vi "Insert SubPanl.vi"(8 "error in (no error)":errorcluster, 10 "VI Ref":refnum<vi>, 11 "Subpanel Ref":refnum<vi>) -> (0 "error out":errorcluster)   [LabVIEW 2021, in "Model.lvlib"]
doc: "<b>Note:</b> This VI was modified by the <b>Validate DQMH Module</b> tool to turn off automatic error handling."
uses:
  Model/Model.lvlib
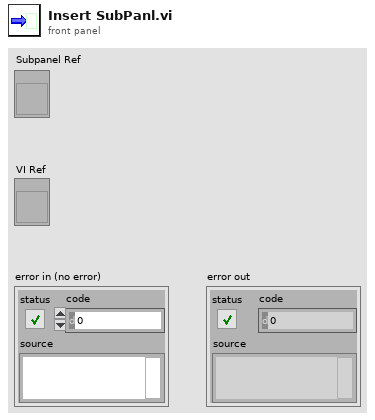
[diagram p1: front panel]
types:
  T1 = enum32{"Invalid", "Standard", "Closed", "Hidden", "Minimized", "Maximized"}
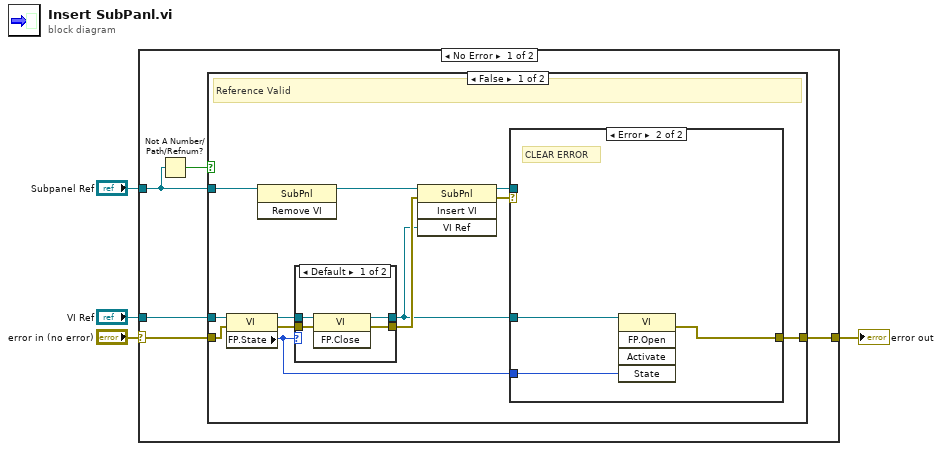
[diagram p0: block diagram]
diagram:
  n1 = case shown="No Error" "error in (no error)" {
    selector: "error in (no error)" -> [w8 w33]
    tunnel: "VI Ref" -> [w9 _]
    tunnel: "Subpanel Ref" -> [w5 _]
    tunnel: [w7 w33] -> w1
    frame No Error {
      n2 = Not A Number/Path/Refnum?(number/path/refnum=w5) -> (NaN/Path/Refnum?=w6:bool)
      n3 = case shown="False" w6 {
        tunnel: w9 -> [w21 _]
        tunnel: w8 -> [w13 w32]
        tunnel: [w12 w32] -> w7
        tunnel: w5 -> [w11 _]
        frame False {
          # "Reference Valid"
          n4 = property class="VI"(reference=w21, error in=w13) -> (reference out=w20:refnum<vi>, error out=w19:errorcluster, "FP.State"=w14:T1)
          n5 = invoke class="SubPnl" method="Remove VI"(reference=w11) -> (reference out=w10:refnum<vi>)  [unwired: 2 in, 2 out]
          n6 = case shown="Default" w14 {
            tunnel: w20 -> [w25 w27]
            tunnel: w19 -> [w24 w26]
            tunnel: [w23 w27] -> w15
            tunnel: [w22 w26] -> w18
            frame Default {
              n7 = invoke class="VI" method="FP.Close"(reference=w25, error in=w24) -> (reference out=w23:refnum<vi>, error out=w22:errorcluster)  [unwired: 1 in, 1 out]
            }
            frame "Closed" {
            }
          }
          n8 = invoke class="SubPnl" method="Insert VI"(reference=w10, error in=w18, "VI Ref"=w15) -> (reference out=w16:refnum<vi>, error out=w17:errorcluster)  [unwired: 1 in, 2 out]
          n9 = case shown="Error" w17 {
            selector: w17 -> [w28 _]
            tunnel: w16 -> [_ _]
            tunnel: w15 -> [_ w31]
            tunnel: w14 -> [_ w30]
            tunnel: [w28 w29] -> w12
            frame No Error {
            }
            frame Error {
              # "CLEAR ERROR"
              n10 = invoke class="VI" method="FP.Open"(reference=w31, "State"=w30) -> (error out=w29:errorcluster)  [unwired: 3 in, 4 out]
            }
          }
        }
        frame True {
          # "Not a reference"
        }
      }
    }
    frame Error {
    }
  }
  "error out" <- w1
